vi "Control - Diesel - EGR Valve Mass Flow.vi"(11 "Control Inputs":T1={"Engine Speed [RPM]"=0.0, "Engine Status"=enum."STALLED", "Load Control \nMode"=enum."High-Idle Governor", "dt(s)"=0.0, "Number of Cylinders"=0, "Engine Displacement [cc]"=0.0, "StoichAFR"=0.0, "Q.LHV Fuel [kJ/kg]"=0.0, "BattV PSU [V]"=0.0, "12V PSU [V]"=0.0, "5V PSU [V]"=0.0, "Pedal Position [%]"=0.0, "Oil Pressure [kPa]"=0.0, "Oil Temp [C]"=0.0, "Oil Level [%]"=0.0, "Engine Coolant Temp (ECT) [C]"=0.0, "Engine Coolant Pressure [kPa]"=0.0, "Rail Pressure [bar]"=0.0, "Fuel Pressure [kPa]"=0.0, "Fuel Temp [C]"=0.0, "Vacuum Pressure [kPa]"=0.0, "Throttle Position [%]"=0.0, "Cam1 Advance [CAD]"=0.0, "Cam2 Advance [CAD]"=0.0, "CA50 Control Output [CAD]"=[], "CA50 Control Output Valid"=[], "Intake Air Temp (IAT) [C]"=0.0, "Barometric Air Pressure [kPa]"=0.0, "Intake Air Rel. Humidity [%]"=0.0, "Mass Air Flow (MAF) [kg/hr]"=0.0, "Turbo Inlet Air Pressure [kPa]"=0.0, "Turbo Inlet Air Temp [C]"=0.0, "Turbo Outlet Air Pressure [kPa]"=0.0, "Turbo Outlet Air Temp [C]"=0.0, "CAC Outlet Pressure [kPa]"=0.0, "CAC Outlet Temp [C]"=0.0, "Intake Manifold Pressure (MAP) [kPa]"=0.0, "Intake Manifold Temp (MAT) [C]"=0.0, "Exhaust Manifold Pressure [kPa]"=0.0, "Exhaust Manifold Temp [C]"=0.0, "HighP EGR Cooler Outlet Pressure [kPa]"=0.0, "HighP EGR Cooler Outlet Temp [C]"=0.0, "HighP EGR Differential Pressure [kPa]"=0.0, "HighP EGR Valve Position [%]"=0.0, "Turbo Outlet Exhaust Pressure [kPa]"=0.0, "Turbo Outlet Exhaust Temp [C]"=0.0, "VGT Position 1 [%]"=0.0, "VGT Position 2 [%]"=0.0, "Turbo Speed 1 [RPM]"=0.0, "Turbo Speed 2 [RPM]"=0.0, "LowP EGR Differential Pressure [kPa]"=0.0, "LowP EGR Valve Position [%]"=0.0, "UEGO1Lambda"=0.0, "UEGO1_Hot"=FALSE, "UEGO2Lambda"=0.0, "UEGO2_Hot"=FALSE} {"CA50 Control Output [CAD]" format="%.2f"; "Turbo Speed 2 [RPM]" format="%.2f"; "LowP EGR Valve Position [%]" format="%.2f"; "CAC Outlet Pressure [kPa]" format="%#_6f"; "UEGO2Lambda" format="%.2f"; "UEGO1Lambda" format="%.2f"; "Intake Manifold Pressure (MAP) [kPa]" format="%#_6f"}) -> (0 "EGR Mass Flow [kg/hr]":sgl)   [LabVIEW 2015, in "ECS-RT.lvlib"]
uses:
  ECS-RT.lvlib
  Typedefs/Control Inputs/Control Inputs.ctl
  Typedefs/EPT/Engine Status.ctl
  Typedefs/MISC/Load Control Mode.ctl
  ECS-Shared.lvlib
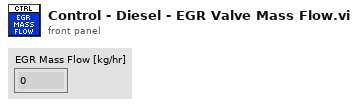
[diagram p1: front panel]
types:
  T1 = typedef "ECS-Shared.lvlib/Control Inputs.ctl" = cluster{"Engine Speed [RPM]":sgl, "Engine Status":T2, "Load Control \nMode":T3, "dt(s)":sgl, "Number of Cylinders":u8, "Engine Displacement [cc]":sgl, "StoichAFR":sgl, "Q.LHV Fuel [kJ/kg]":sgl, "BattV PSU [V]":sgl, "12V PSU [V]":sgl, "5V PSU [V]":sgl, "Pedal Position [%]":sgl, "Oil Pressure [kPa]":sgl, "Oil Temp [C]":sgl, "Oil Level [%]":sgl, "Engine Coolant Temp (ECT) [C]":sgl, "Engine Coolant Pressure [kPa]":sgl, "Rail Pressure [bar]":sgl, "Fuel Pressure [kPa]":sgl, "Fuel Temp [C]":sgl, "Vacuum Pressure [kPa]":sgl, "Throttle Position [%]":sgl, "Cam1 Advance [CAD]":sgl, "Cam2 Advance [CAD]":sgl, "CA50 Control Output [CAD]":sgl[], "CA50 Control Output Valid":bool[], "Intake Air Temp (IAT) [C]":sgl, "Barometric Air Pressure [kPa]":sgl, "Intake Air Rel. Humidity [%]":sgl, "Mass Air Flow (MAF) [kg/hr]":sgl, "Turbo Inlet Air Pressure [kPa]":sgl, "Turbo Inlet Air Temp [C]":sgl, "Turbo Outlet Air Pressure [kPa]":sgl, "Turbo Outlet Air Temp [C]":sgl, "CAC Outlet Pressure [kPa]":sgl, "CAC Outlet Temp [C]":sgl, "Intake Manifold Pressure (MAP) [kPa]":sgl, "Intake Manifold Temp (MAT) [C]":sgl, "Exhaust Manifold Pressure [kPa]":sgl, "Exhaust Manifold Temp [C]":sgl, "HighP EGR Cooler Outlet Pressure [kPa]":sgl, "HighP EGR Cooler Outlet Temp [C]":sgl, "HighP EGR Differential Pressure [kPa]":sgl, "HighP EGR Valve Position [%]":sgl, "Turbo Outlet Exhaust Pressure [kPa]":sgl, "Turbo Outlet Exhaust Temp [C]":sgl, "VGT Position 1 [%]":sgl, "VGT Position 2 [%]":sgl, "Turbo Speed 1 [RPM]":sgl, "Turbo Speed 2 [RPM]":sgl, "LowP EGR Differential Pressure [kPa]":sgl, "LowP EGR Valve Position [%]":sgl, "UEGO1Lambda":sgl, "UEGO1_Hot":bool, "UEGO2Lambda":sgl, "UEGO2_Hot":bool}
  T2 = typedef "ECS-Shared.lvlib/Engine Status.ctl" = enum16{"STALLED", "CRANKING", "RUNNING"}
  T3 = typedef "ECS-Shared.lvlib/Load Control Mode.ctl" = enum16{"No Governor", "Low-Idle Governor", "High-Idle Governor"}
  T4 = cluster{"Valve Inlet Pressure [kPa]":sgl, "Valve Outlet Pressure [kPa]":sgl, "Valve Inlet Temp [C]":sgl, "Valve Position [%Open]":sgl, "Valve Diameter [m]":sgl, "R - Gas constant [J/kg-K]":sgl, "k - Ratio of specific heats":sgl, "Valve Cd":sgl}
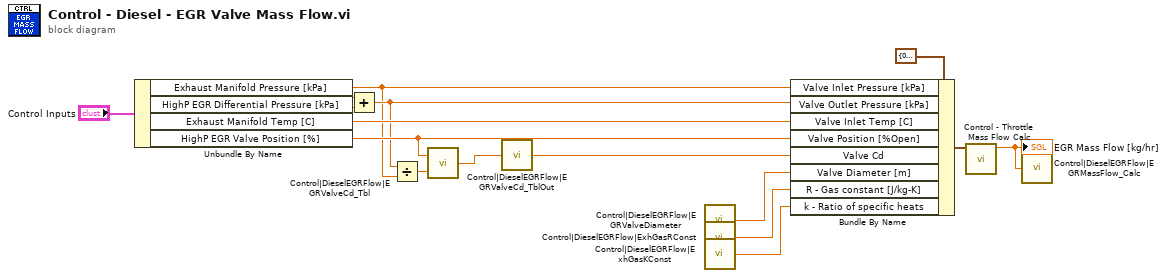
[diagram p0: block diagram]
diagram:
  n1 = Unbundle By Name("Control Inputs") -> ("Exhaust Manifold Pressure [kPa]"=w4:sgl, "HighP EGR Differential Pressure [kPa]"=w13:sgl, "Exhaust Manifold Temp [C]"=w12:sgl, "HighP EGR Valve Position [%]"=w7:sgl)
  n2 = Add(x=w4, y=w13) -> (x+y=w5:sgl)
  n3 = Divide(x=w5, y=w4) -> (x/y=w6:sgl)
  n4 = call "Control|DieselEGRFlow|EGRValveCd_Tbl"("Y Index"=w6, "X Index"=w7) -> ("Z"=w3:sgl)
  n5 = call "Control|DieselEGRFlow|EGRValveCd_TblOut"("Value"=w3) -> ()
  n6 = call "Control|DieselEGRFlow|EGRValveDiameter"() -> ("Value"=w8:sgl)
  n7 = call "Control|DieselEGRFlow|ExhGasRConst"() -> ("Value"=w10:sgl)
  n8 = call "Control|DieselEGRFlow|ExhGasKConst"() -> ("Value"=w9:sgl)
  n9 = Bundle By Name(cluster=T4 {"Valve Inlet Pressure [kPa]"=0.0, "Valve Outlet Pressure [kPa]"=0.0, "Valve Inlet Temp [C]"=0.0, "Valve Position [%Open]"=0.0, "Valve Diameter [m]"=0.0, "R - Gas constant [J/kg-K]"=289.0, "k - Ratio of specific heats"=1.4, "Valve Cd"=0.0} ("Inputs"), "Valve Inlet Pressure [kPa]"=w4, "Valve Outlet Pressure [kPa]"=w5, "Valve Inlet Temp [C]"=w12, "Valve Position [%Open]"=w7, "Valve Cd"=w3, "Valve Diameter [m]"=w8, "R - Gas constant [J/kg-K]"=w10, "k - Ratio of specific heats"=w9) -> (w11:T4)
  n10 = call "Control - Throttle Mass Flow Calc.vi"("Inputs"=w11) -> ("Throttle Mass Flow [kg/hr]"=w1:sgl)  [unwired: 10 in]
  "EGR Mass Flow [kg/hr]" <- w1
  n11 = call "Control|DieselEGRFlow|EGRMassFlow_Calc"("Value"=w1) -> ()
